vi "Actor Core.vi"(8 "error in":errorcluster, 11 "Chat Room Model in":refnum<class "Chat Room Model.lvclass">) -> (0 "error out":errorcluster, 3 "Actor out":refnum<class "Actor.lvclass">)   [LabVIEW 2018, in "Chat Room Model.lvlib" / "Chat Room Model.lvclass"]
doc: "(<B>Filename</B>: Actor Framework.lvlib:Actor.lvclass:Actor Core.vi)\n\nReceives messages to the actor, reacts to them, and initiates any error handling that may shut the actor down.\n\nDescendant classes may override this VI to append parallel tasks for the actor to complete while it handles messages. Overrides use the Call Parent Method node."
uses:
  Chat Room Model.lvclass
  C:/Program Files (x86)/National Instruments/LabVIEW 2018/vi.lib/ActorFramework/Actor/Actor.lvclass
  <vilib>/ActorFramework/Actor/Actor.lvclass
  Chat Room Controller/Chat Room Controller/Chat Room Controller.lvclass
  Chat Room Model.lvclass/Chat Room Model.ctl
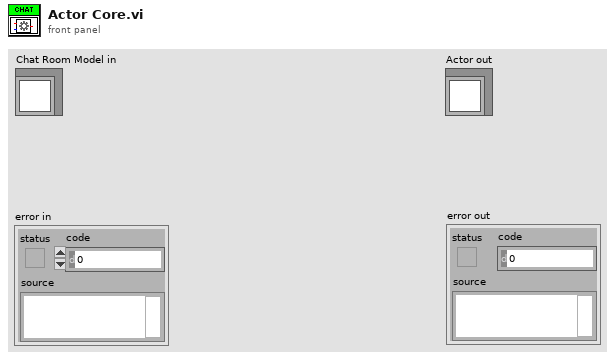
[diagram p1: front panel]
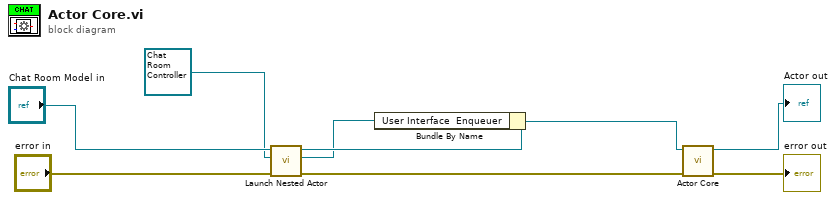
[diagram p0: block diagram]
diagram:
  n1 = call <vilib>:"Launch Nested Actor.vi"("error in (no error)"="error in", "Nested Actor"=refnum<class "Chat Room Controller.lvclass"> refnum ("Chat Room Controller.lvlib:Chat Room Controller.lvclass"), "Caller Actor in"="Chat Room Model in") -> ("error out"=w5:errorcluster, "Nested Actor's Enqueuer"=w1:refnum<class "Message Enqueuer.lvclass">, "Caller Actor out"=w3:refnum<class "Chat Room Model.lvclass">)  [unwired: 6 in]
  n2 = Bundle By Name(cluster=w3, "User Interface  Enqueuer"=w1) -> (w2:refnum<class "Chat Room Model.lvclass">)
  n3 = call-parent "Actor Core.vi"("error in"=w5, "Actor in"=w2) -> ("error out"=→"error out":errorcluster, "Actor out"=→"Actor out":refnum<class "Actor.lvclass">)  [unwired: 8 in]
